vi "Generic command handler.vi"(8 "error in (no error)":errorcluster, 10 "Message in":refnum<class "GenericMessage.lvclass">, 11 "Chat in":refnum<class "Chat.lvclass">) -> (0 "error out":errorcluster, 2 "value":string, 3 "Chat out":refnum<class "Chat.lvclass">)   [LabVIEW 2012, in "Chat.lvclass"]
doc: "The generic_command_handler processes the command 'generic'. Commands which are not part of the predefined list of commands fall under the 'generic' command for special activity."
uses:
  Chat.lvclass
  <vilib>/Distrio/Murmex/GenericMessage/GenericMessage.lvclass
  <vilib>/Distrio/Murmex/Murmex/Murmex.lvclass
panel:
  # "This method is called when the GENERIC\ntrigger is sent. \n\nOverride this method when your component needs to\nrespond to this trigger. \n\nCall parent for proper implementation"
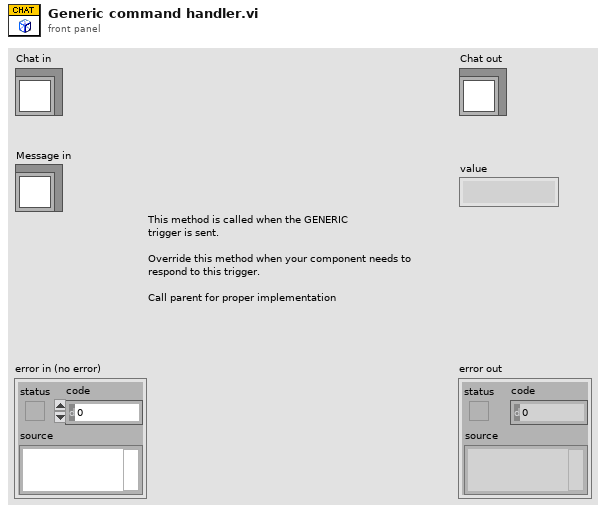
[diagram p1: front panel]
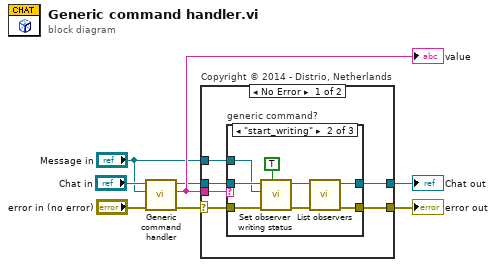
[diagram p0: block diagram]
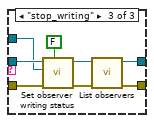
[diagram p3: hidden frame]
diagram:
  n1 = call-parent "Generic command handler.vi"("error in (no error)"="error in (no error)", "Message in"="Message in", "Murmex in"="Chat in") -> ("error out"=w6:errorcluster, "value"=w4:string, "Murmex out"=w2:refnum<class "Chat.lvclass">)  [unwired: 6 in]
  "value" <- w4
  n2 = case "Copyright © 2014 - Distrio, Netherlands" shown="No Error" w6 {
    selector: w6 -> [w12 w34]
    tunnel: [w13 w34] -> w5
    tunnel: w4 -> [w14 _]
    tunnel: "Message in" -> [w11 _]
    tunnel: w2 -> [w10 w33]
    tunnel: [w9 w33] -> w1
    frame No Error {
      n3 = case "generic command?" shown="\"start_writing\"" w14 {
        tunnel: [w16 w17 w27] -> w13
        tunnel: w12 -> [w16 w24 w32]
        tunnel: w11 -> [_ w22 w30]
        tunnel: w10 -> [w15 w23 w31]
        tunnel: [w15 w18 w25] -> w9
        frame Default {
        }
        frame "start_writing" {
          n4 = call "Set observer writing status.vi"("writing"=TRUE, "error in (no error)"=w24, "Message in"=w22, "Chat in"=w23) -> ("error out"=w20:errorcluster, "Chat out"=w19:refnum<class "Chat.lvclass">)  [unwired: 6 in]
          n5 = call "List observers.vi"("error in (no error)"=w20, "Chat in"=w19) -> ("error out"=w17:errorcluster, "Chat out"=w18:refnum<class "Chat.lvclass">)  [unwired: 8 in]
        }
        frame "stop_writing" {
          n6 = call "Set observer writing status.vi"("writing"=FALSE, "error in (no error)"=w32, "Message in"=w30, "Chat in"=w31) -> ("error out"=w28:errorcluster, "Chat out"=w26:refnum<class "Chat.lvclass">)  [unwired: 6 in]
          n7 = call "List observers.vi"("error in (no error)"=w28, "Chat in"=w26) -> ("error out"=w27:errorcluster, "Chat out"=w25:refnum<class "Chat.lvclass">)  [unwired: 8 in]
        }
      }
    }
    frame Error {
    }
  }
  "error out" <- w5
  "Chat out" <- w1
